vi "UVer.vi"() -> ()   [LabVIEW 2012]
panel:
  in  "stop":bool
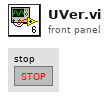
[diagram p1: front panel]
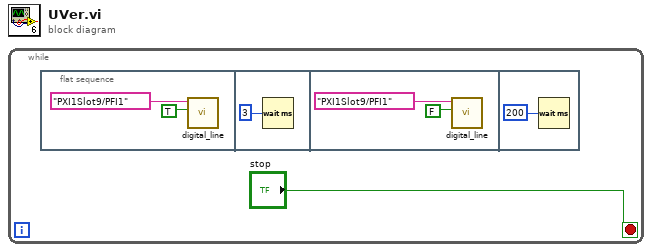
[diagram p0: block diagram]
diagram:
  n1 = while {
    stop <- "stop" stop-if-true
    n2 = flat-sequence {
      frame #0 {
        n3 = call "digital_line.vi"("Boolean"=TRUE, "lines"=tag "PXI1Slot9/PFI1") -> ()  [unwired: 5 in, 1 out]
      }
      frame #1 {
        n4 = Wait (ms)(milliseconds to wait=u32 3) -> ()  [unwired: 1 out]
      }
      frame #2 {
        n5 = call "digital_line.vi"("Boolean"=FALSE, "lines"=tag "PXI1Slot9/PFI1") -> ()  [unwired: 5 in, 1 out]
      }
      frame #3 {
        n6 = Wait (ms)(milliseconds to wait=u32 200) -> ()  [unwired: 1 out]
      }
    }
  }
